vi "LSX Get Slide.vi"(7 "mode":i32, 8 "error in (no error)":errorcluster, 9 "slot":i32, 10 "maga":i32, 11 "lLSID":i32) -> (0 "error out":errorcluster, 3 "function return":i32)   [LabVIEW 2018, in "Tango.lvlib"]
doc: "TANGOAPI int TANGOCALL LSX_GetSlide (int lLSID, int maga, int slot, int mode);"
uses:
  Tango.lvlib
  SubVIs/Tango_DLL.dll
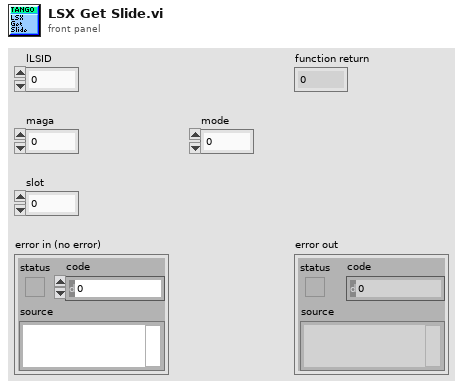
[diagram p1: front panel]
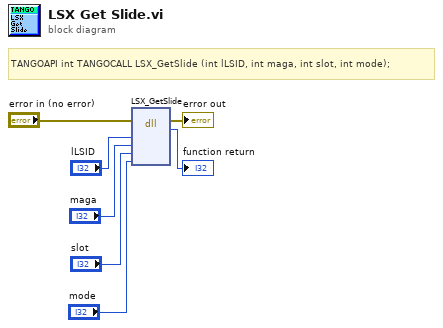
[diagram p0: block diagram]
diagram:
  # "TANGOAPI int TANGOCALL LSX_GetSlide (int lLSID, int maga, int slot, int mode);"
  n1 = dll-call lib="C:/Users/Familie/Documents/LabviewIX81/lib/TANGO Stage/SubVIs/Tango_DLL.*" fn="LSX_GetSlide"(error in="error in (no error)", "lLSID"="lLSID", "maga"="maga", "slot"="slot", "mode"="mode") -> (error out=→"error out":errorcluster, →"function return":i32)  [unwired: 6 in, 1 out]
